vi "Paths.vi"(10 "Project":string, 11 "Max Status Logs (-1: unlimited)":i32=-1) -> (2 "Config Path":path, 3 "Status Path":path)   [LabVIEW 2015, in "Endigit.lvlib"]
doc: "Provides paths for Status.vi and Configit based on the project name. Paths are both in the Public Documents in Windows. The config path points to the specific ini file while the status path points to a new file each time the application is run. Any non-existing folders are created. If a number is provided for \"Max Status Logs\" then this VI will delete all but the newest however many are specified.\n\nAuthored by Robert C. Mortensen\nrobert@endigit.com\n\nCopyright (c) 2015, Endigit, Inc."
uses:
  Endigit.lvlib
  <vilib>/Utility/sysdir.llb/System Directory Type.ctl
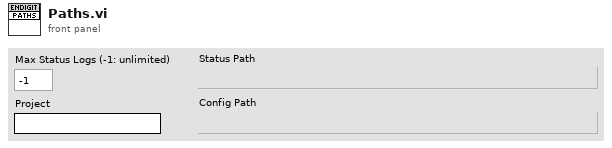
[diagram p1: front panel]
types:
  T1 = typedef "System Directory Type.ctl" = i32
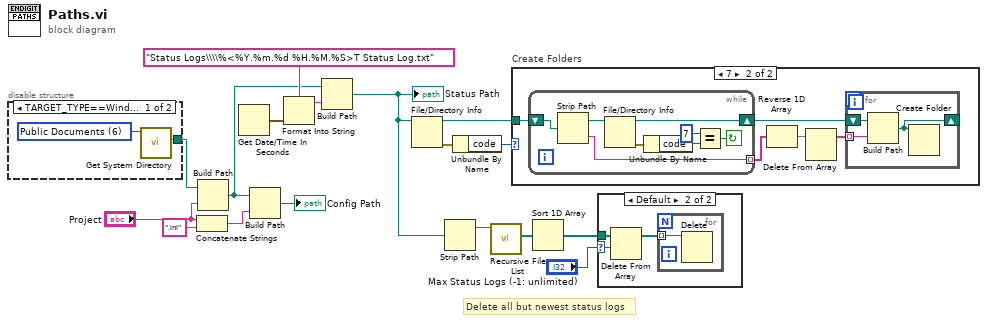
[diagram p0: block diagram]
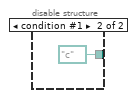
[diagram p3: hidden frame]
diagram:
  # "Delete all but newest status logs"
  n1 = disable-structure shown="TARGET_TYPE==Windows, Default" {
    disable-tunnel: [w18 path "c:/" ("system directory")] -> w7
    frame condition #0 (active) {
      w19 = T1 6 items=["User Home"=0, "User Desktop"=1, "User Documents"=2, "User Application Data"=3, "User Preferences"=4, "User Temporary"=5, "Public Documents"=6, "Public Application Data"=7, "Public Preferences"=8, "Public Cache"=13, "System Core Libraries"=9, "System Installed Libraries"=10, "Application Files"=11, "Boot Volume Root"=12] ("system directory type")
      n2 = call <vilib>:"Get System Directory.vi"("system directory type"=w19) -> ("system directory"=w18:path)  [unwired: 10 in]
    }
    frame condition #1 {
    }
  }
  n3 = Concatenate Strings("Project", ".ini" ("File Extension (.ini)")) -> (w17:string)
  n4 = Build Path(base path=w7, name or relative path="Project") -> (appended path=w12:path)
  n5 = Get Date/Time In Seconds() -> (seconds since 1Jan1904=w14:timestamp)
  n6 = Build Path(base path=w12, name or relative path=w17) -> (appended path=→"Config Path":path)
  n7 = Format Into String(format string="Status Logs\\\\%<%Y.%m.%d %H.%M.%S>T Status Log.txt", w14) -> (resulting string=w13:string)  [unwired: 2 in, 1 out]
  n8 = Build Path(base path=w12, name or relative path=w13) -> (appended path=w3:path)
  "Status Path" <- w3
  n9 = File/Directory Info(path=w3) -> (path out=w8:path, error out=w10:errorcluster)  [unwired: 1 in, 5 out]
  n10 = Strip Path(path=w3) -> (stripped path=w4:path)  [unwired: 1 out]
  n11 = Unbundle By Name(w10) -> ("code"=w9:i32)
  n12 = call <vilib>:"Recursive File List.vi"("Folder Path"=w4) -> ("All Files in Dir"=w5:path[])  [unwired: 6 in, 4 out]
  n13 = case "Create Folders" shown="7" w9 {
    tunnel: w8 -> [_ w23]
    frame Default {
    }
    frame 7 {
      n14 = while {
        shift-right: [w29] -> w24
        shift-left: w23 -> [w36]
        tunnel: [w30] -> w25 mode=indexing
        stop <- w31 continue-if-true
        n15 = Strip Path(path=w36) -> (stripped path=w35:path, name=w30:string)
        n16 = File/Directory Info(path=w35) -> (path out=w29:path, error out=w34:errorcluster)  [unwired: 1 in, 5 out]
        n17 = Unbundle By Name(w34) -> ("code"=w33:i32)
        n18 = Equal?(x=7 ("y"), y=w33) -> (x = y?=w31:bool)
      }
      n19 = Reverse 1D Array(array=w25) -> (reversed array=w22:string[])
      n20 = Delete From Array(array=w22) -> (array with subset deleted=w21:string[])  [unwired: 2 in, 1 out]
      n21 = for {
        shift-right: [w26] -> _
        shift-left: w24 -> [w28]
        tunnel: w21 -> [w27] mode=indexing
        n22 = Build Path(base path=w28, name or relative path=w27) -> (appended path=w26:path)
        n23 = Create Folder(path (use dialog)=w26) -> ()  [unwired: 2 in, 3 out]
      }
    }
  }
  n24 = Sort 1D Array(array=w5) -> (sorted array=w6:path[])
  n25 = case shown="Default" "Max Status Logs (-1: unlimited)" {
    selector: "Max Status Logs (-1: unlimited)" -> [_ w37]
    tunnel: w6 -> [_ w38]
    frame ..0 {
    }
    frame Default {
      n26 = Delete From Array(array=w38, length=w37) -> (array with subset deleted=w39:path[])  [unwired: 1 in, 1 out]
      n27 = for {
        tunnel: w39 -> [w40] mode=indexing
        n28 = Delete(path (use dialog)=w40) -> ()  [unwired: 1 in, 6 out]
      }
    }
  }
